vi "lvProfileRename.vi"(6 "error in (no error)":errorcluster, 7 "newName":string, 8 "oldName":string, 9 "Path to Python.exe":path=path "C:/ProgramData/Anaconda3/python.exe") -> (0 "error out":errorcluster, 3 "Raw Python String Output":string)   [LabVIEW 2017]
panel:
  out "Standard Error":string
  out "Return Code":i32
  # "1. Inputs - Set before running VI"
  # "2. Outputs"
  # "3. Errors - Both Standard and LabVIEW"
  # "A + B ="
  # "This VI sends inputs to a simple Python script, and returns its output.\n\nSee block diagram for code and comments"
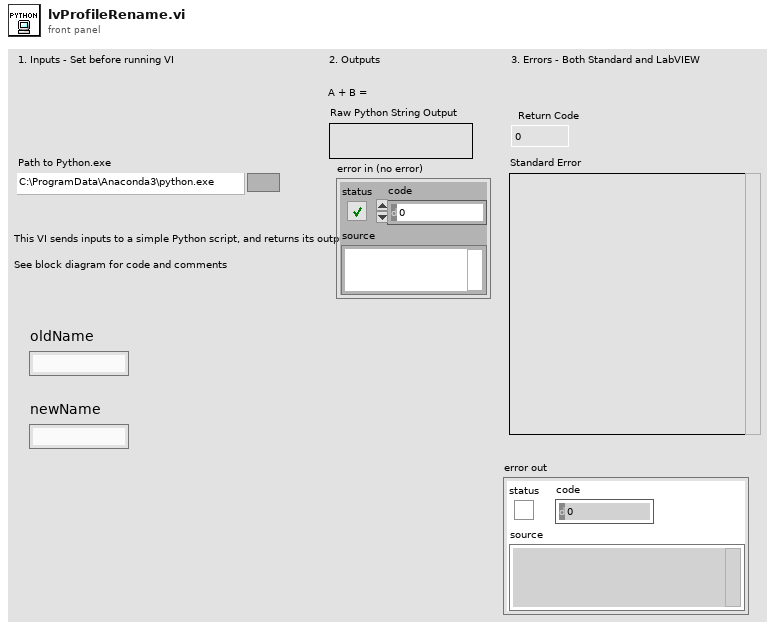
[diagram p1: front panel]
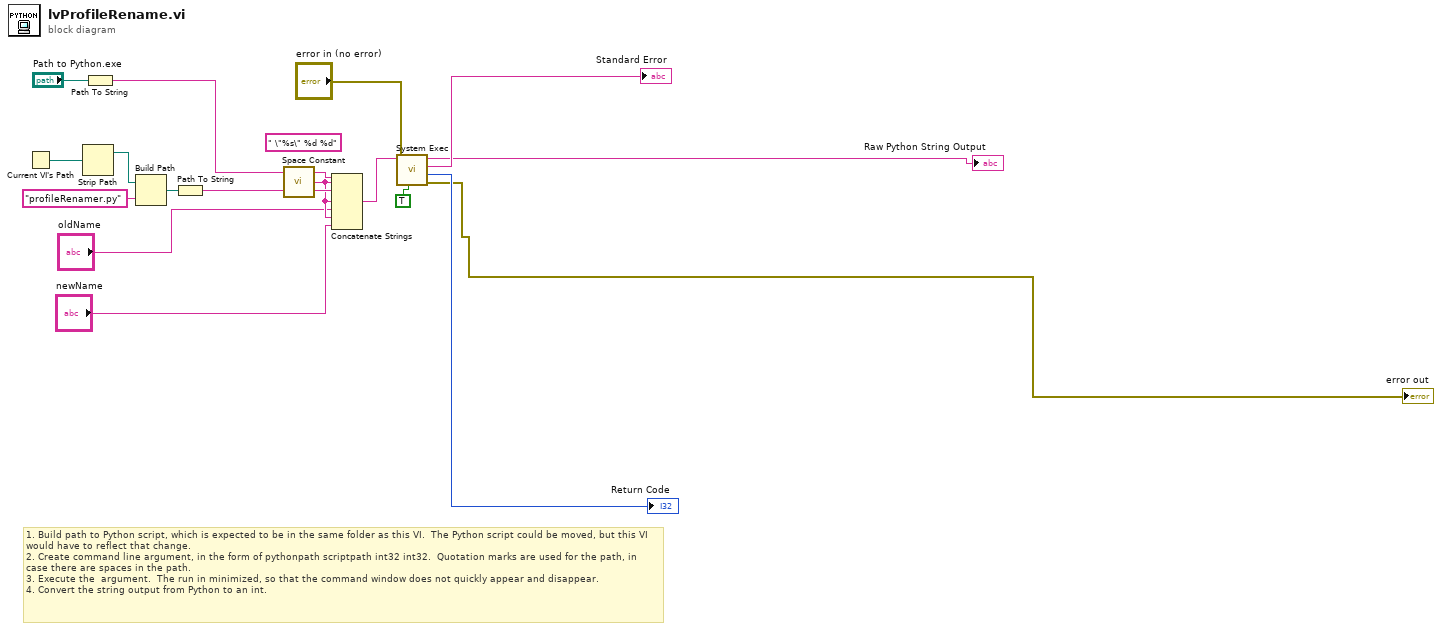
[diagram p0: block diagram]
diagram:
  (unwired) " \"%s\" %d %d" ("format string")
  # "1. Build path to Python script, which is expected to be in the same folder as this VI.  The Python script could be moved, but this VI would have to reflect that change.\n2. Create command line argument, in the form of pythonpath scriptpath int32 int32.  Quotation marks are used for the path, in case there are spaces in the path.\n3. Execute the  argument.  The run in minimized, so that the command window does not quickly appear and disappear.\n4. Convert the string output from Python to an int."
  n1 = Current VI's Path() -> (path=w12:path)
  n2 = Strip Path(path=w12) -> (stripped path=w10:path)  [unwired: 1 out]
  n3 = Path To String(path="Path to Python.exe") -> (string=w7:string)
  n4 = Build Path(base path=w10, name or relative path="profileRenamer.py" ("Path to Function")) -> (appended path=w13:path)
  n5 = Path To String(path=w13) -> (string=w8:string)
  n6 = call <vilib>:"Space Constant.vi"() -> ("String"=w3:string)
  n7 = Concatenate Strings(w7, w3, w8, w3, "oldName", w3, "newName") -> (w9:string)
  n8 = call <vilib>:"System Exec.vi"("run minimized? (F)"=TRUE, "error in (no error)"="error in (no error)", "command line"=w9) -> ("error out"=→"error out":errorcluster, "return code"=→"Return Code":i32, "standard error"=→"Standard Error":string, "standard output"=→"Raw Python String Output":string)  [unwired: 5 in]
